vi "DataPath.vi"(1 "name":string) -> (0 "path":path)   [LabVIEW 2014]
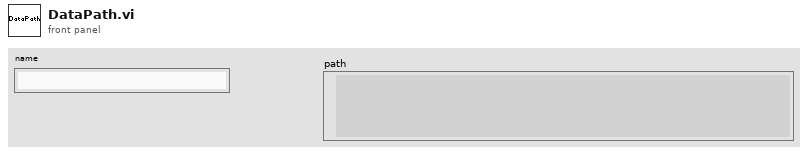
[diagram p1: front panel]
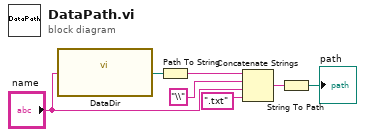
[diagram p0: block diagram]
diagram:
  n1 = call "DataDir.vi"("name"="name") -> ("path"=w3:path)
  n2 = Path To String(path=w3) -> (string=w2:string)
  n3 = Concatenate Strings(w2, "\\" ("string"), "name", ".txt" ("string")) -> (w6:string)
  n4 = String To Path(string=w6) -> (path=→"path":path)
